vi "Modbus_Get_Status_list.vi"(11 "register values":u16[](array[numeric])) -> (1 "Boolean":bool, 2 "Boolean 2":bool, 3 "Boolean array":bool[](array[boolean]))   [LabVIEW 2020]
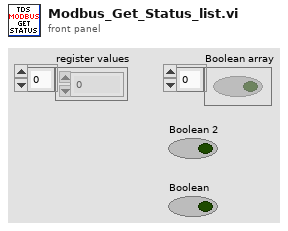
[diagram p1: front panel]
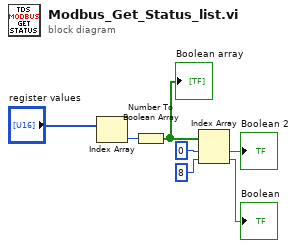
[diagram p0: block diagram]
diagram:
  n1 = Index Array(array="register values") -> (element=w2:u16)  [unwired: 1 in]
  n2 = Number To Boolean Array(number=w2) -> (Boolean array=w3:bool[])
  "Boolean array" <- w3
  n3 = Index Array(array=w3, index #1=0 ("index"), index #2=8 ("index")) -> (element #1=→"Boolean 2":bool, element #2=→"Boolean":bool)
